vi "Create from string.vi"(11 "address string":string) -> (3 "address":refnum<class "MacOS Network Address.lvclass">)   [LabVIEW 2020, in "NI_WFCN.lvlib" / "MacOS Network Address.lvclass"]
doc: "Create a MacOS network address from a string. This does no parsing, it just blindly accepts whatever is passed in."
uses:
  <vilib>/net/WFCN/Addressing/MacOS Network Address/MacOS Network Address.lvclass
  <vilib>/net/WFCN/Addressing/MacOS Network Address/MacOS Network Address.lvclass/MacOS Network Address.ctl
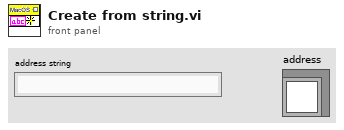
[diagram p1: front panel]
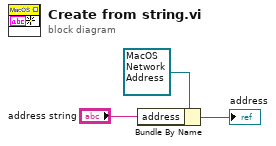
[diagram p0: block diagram]
diagram:
  n1 = Bundle By Name(cluster=refnum<class "MacOS Network Address.lvclass"> refnum ("MacOS Network Address in"), "address"="address string") -> (→"address":refnum<class "MacOS Network Address.lvclass">)
